vi "BadDeploymentCountGV.vi"(8 "error in (no error)":errorcluster, 9 "SetBadDeployments":dbl, 10 "GetOrSet":enum16{"Get", "Set"}(ring)) -> (0 "error out":errorcluster, 2 "BadDeployCount":dbl)   [LabVIEW 2016]
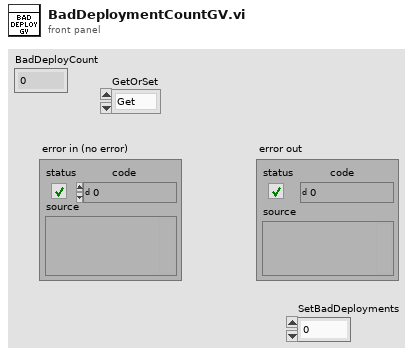
[diagram p1: front panel]
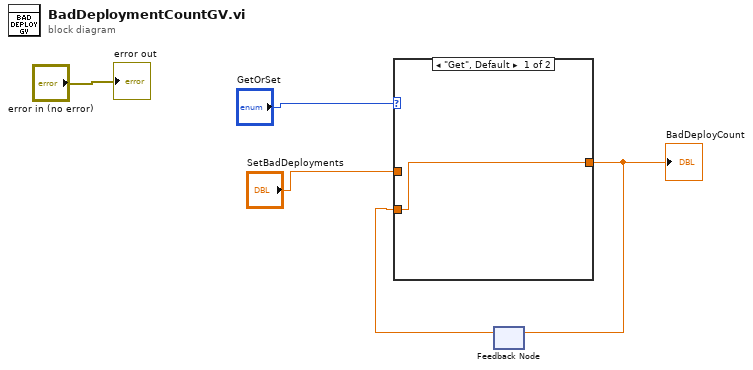
[diagram p0: block diagram]
diagram:
  n1 = feedback #1() -> (w2:dbl)  [unwired: 1 in]
  n2 = case shown="\"Get\", Default" "GetOrSet" {
    tunnel: "SetBadDeployments" -> [_ w7]
    tunnel: [w6 w7] -> w3
    tunnel: w2 -> [w6 _]
    frame "Get", Default {
    }
    frame "Set" {
    }
  }
  "BadDeployCount" <- w3
  n3 = feedback-in #1(w3) -> ()
  "error out" <- "error in (no error)"
